vi "EXO_SignalRecord1.vi"(0 "LN2 Level_Dewar 1":dbl, 1 "Xe Level":dbl, 2 "Pressure 3":dbl, 3 "Pressure 2":dbl, 5 "Flow Speed":dbl, 7 "LN2 Level_Dewar 2":dbl, 8 "Pressure 1":dbl, 9 "Temperature 3_Thermocouple":dbl, 10 "Temperature 2_DT":dbl, 11 "Temperature 1_PT":dbl) -> (6 "output cluster":T1)   [LabVIEW 2012]
panel:
  out "current time":timestamp
  in  "stop":bool
  # "EXO DatabaseWrite Sub-VI (I)"
  # "Data List\nTemperature: PT, DT, Thermocouple\nPressure: Sensor1, Sensor2, Sensor3\nLevel Measurement: Xe, Liquid Nitrogen 1, Liquid Nitrogen 2\nFlow Speed: MKS"
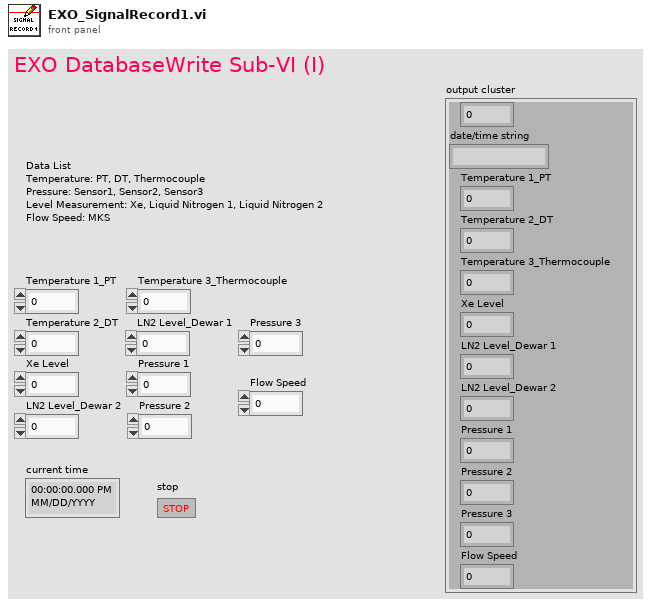
[diagram p1: front panel]
types:
  T1 = cluster{dbl, "date/time string":string, "Temperature 1_PT":dbl, "Temperature 2_DT":dbl, "Temperature 3_Thermocouple":dbl, "Xe Level":dbl, "LN2 Level_Dewar 1":dbl, "LN2 Level_Dewar 2":dbl, "Pressure 1":dbl, "Pressure 2":dbl, "Pressure 3":dbl, "Flow Speed":dbl}
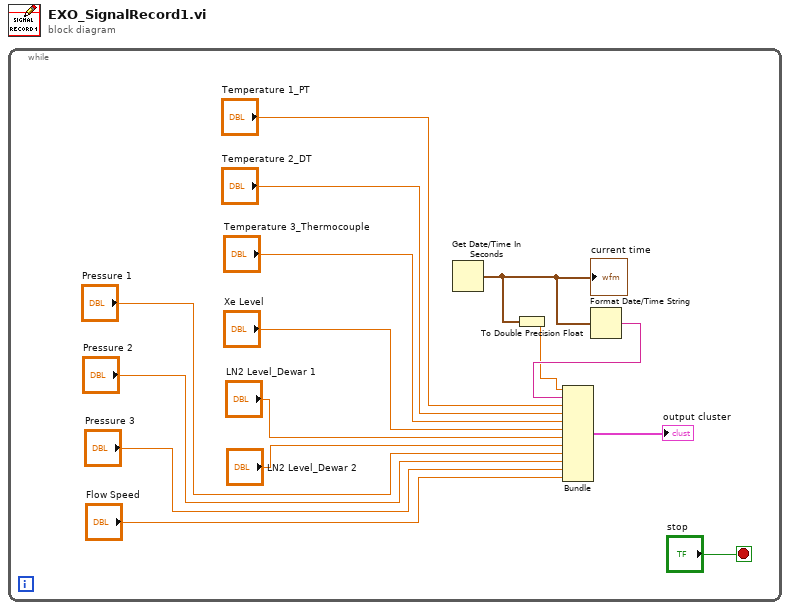
[diagram p0: block diagram]
diagram:
  n1 = while {
    stop <- "stop" stop-if-true
    n2 = Get Date/Time In Seconds() -> (seconds since 1Jan1904=w13:timestamp)
    "current time" <- w13
    n3 = To Double Precision Float(number=w13) -> (double precision float=w12:dbl)
    n4 = Format Date/Time String(seconds (now)=w13) -> (date/time string=w14:string)  [unwired: 2 in]
    n5 = Bundle(w12, "date/time string"=w14, "Temperature 1_PT"="Temperature 1_PT", "Temperature 2_DT"="Temperature 2_DT", "Temperature 3_Thermocouple"="Temperature 3_Thermocouple", "Xe Level"="Xe Level", "LN2 Level_Dewar 1"="LN2 Level_Dewar 1", "LN2 Level_Dewar 2"="LN2 Level_Dewar 2", "Pressure 1"="Pressure 1", "Pressure 2"="Pressure 2", "Pressure 3"="Pressure 3", "Flow Speed"="Flow Speed") -> (→"output cluster":T1)  [unwired: 1 in]
  }
